vi "Path-Move.vi"(6 "Move Time":u32=500, 7 "Maze Display Ref":refnum<vi>, 8 "error in (no error)":errorcluster, 9 "Tile Array":T2[][](array[typedef]), 10 "Start":T1, 11 "Finish":T1) -> (0 "error out":errorcluster)   [LabVIEW 2020]
doc: "<B>Description:</B> Moves a colored tile through the maze.\n\n<B>Date:</B> 06/2019\n<B>Author:</B> Luke Jarocki, Choose Movement Consulting, LLC"
uses:
  Controls/TileColor.ctl
  Controls/Parse-(X,Y).ctl
panel:
  in  "stop":bool
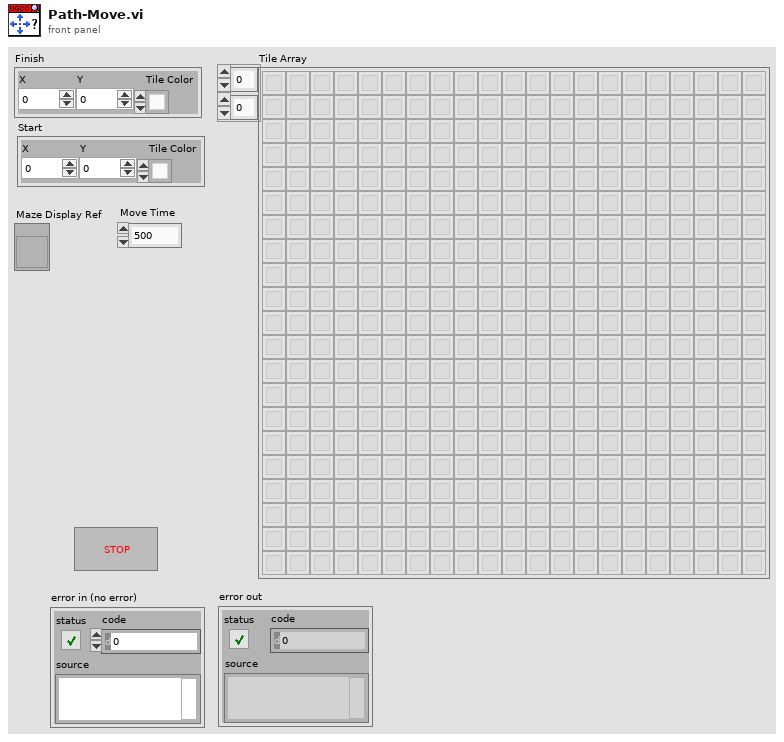
[diagram p1: front panel]
types:
  T1 = typedef "Parse-(X,Y).ctl" = cluster{"X":i32, "Y":i32, "Tile Color":T2}
  T2 = typedef "TileColor.ctl" = u16
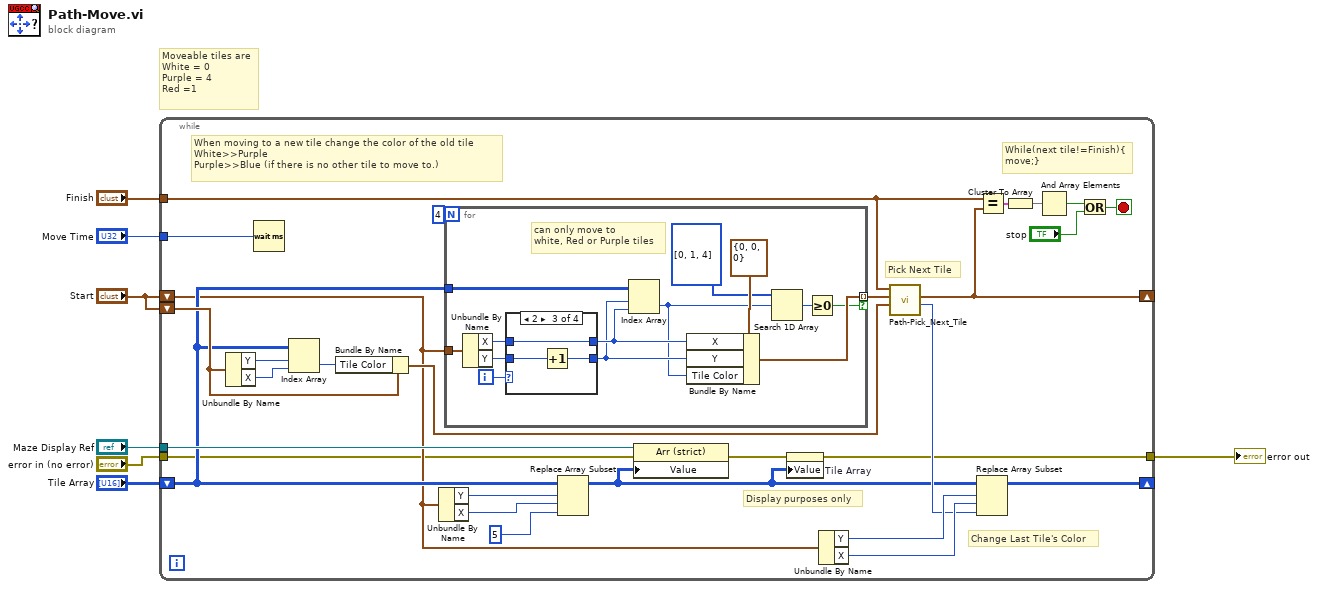
[diagram p0: block diagram]
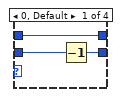
[diagram p2: hidden frame]
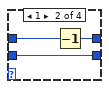
[diagram p3: hidden frame]
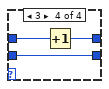
[diagram p4: hidden frame]
diagram:
  # "Moveable tiles are\nWhite = 0\nPurple = 4\nRed =1"
  n1 = while {
    tunnel: "Finish" -> [w15]
    shift-right: [w12] -> _
    shift-left: "Start" -> [w14]
    shift-right: [w33] -> _
    shift-left: "Tile Array" -> [w17]
    shift-left: "Start" -> [w25]
    tunnel: "Maze Display Ref" -> [w21]
    tunnel: "Move Time" -> [w20]
    tunnel: [w8] -> w2
    tunnel: "error in (no error)" -> [w11]
    stop <- w26 stop-if-true
    # "Change Last Tile's Color"
    # "When moving to a new tile change the color of the old tile\nWhite>>Purple\nPurple>>Blue (if there is no other tile to move to.)"
    # "While(next tile!=Finish){\nmove;}"
    # "Display purposes only"
    # "Pick Next Tile"
    n2 = Unbundle By Name(w25) -> ("Y"=w24:i32, "X"=w23:i32)
    n3 = Wait (ms)(milliseconds to wait=w20) -> ()  [unwired: 1 out]
    n4 = Index Array(array=w17, index (row)=w24, index (col)=w23) -> (element=w22:T2)
    n5 = Bundle By Name(cluster=w25, "Tile Color"=w22) -> (w16:T1)
    n6 = Unbundle By Name(w14) -> ("Y"=w19:i32, "X"=w18:i32)
    n7 = for {
      N: 4 -> [_]
      tunnel: w14 -> [w47]
      tunnel: w17 -> [w48]
      tunnel: [w43] -> w35 mode=indexing if=w37
      i -> [w49]
      # "can only move to\nwhite, Red or Purple tiles"
      n8 = Unbundle By Name(w47) -> ("X"=w46:i32, "Y"=w45:i32)
      n9 = case shown="2" w49 {
        tunnel: [w51 w54 w56 w59] -> w42
        tunnel: [w52 w53 w57 w60] -> w41
        tunnel: w46 -> [w51 w55 w56 w61]
        tunnel: w45 -> [w50 w53 w58 w60]
        frame 0, Default {
          n10 = Decrement(x=w50) -> (x-1=w52:i32)
        }
        frame 1 {
          n11 = Decrement(x=w55) -> (x-1=w54:i32)
        }
        frame 2 {
          n12 = Increment(x=w58) -> (x+1=w57:i32)
        }
        frame 3 {
          n13 = Increment(x=w61) -> (x+1=w59:i32)
        }
      }
      n14 = Index Array(array=w48, index (row)=w41, index (col)=w42) -> (element=w39:T2)
      n15 = Bundle By Name(cluster=T1 {"X"=0, "Y"=0, "Tile Color"=0} ("(X,Y)"), "X"=w42, "Y"=w41, "Tile Color"=w39) -> (w43:T1)
      n16 = Search 1D Array(1D array=T2[] [0, 1, 4], element=w39) -> (index of element=w38:i32)  [unwired: 1 in]
      n17 = Greater Or Equal To 0?(x=w38) -> (x >= 0?=w37:bool)
    }
    n18 = Replace Array Subset(array=w17, new element=T2 5 ("new element/subarray"), index (row)=w19, index (col)=w18) -> (w10:T2[][])
    n19 = property class="Arr (strict)"(reference=w21, error in=w11, "Value"=w10) -> (error out=w9:errorcluster)  [unwired: 1 out]
    n20 = property on="Tile Array" class="Arr (strict)"(error in=w9, "Value"=w10) -> (error out=w8:errorcluster)  [unwired: 1 in, 1 out]
    n21 = Unbundle By Name(w14) -> ("Y"=w32:i32, "X"=w31:i32)
    n22 = call "Path-Pick_Next_Tile.vi"("Last Tile"=w16, "Adjacent Tiles"=w35, "Goal"=w15) -> ("Tile"=w13:T2, "New Position"=w12:T1)  [unwired: 7 in]
    n23 = Replace Array Subset(array=w10, new element=w13, index (row)=w32, index (col)=w31) -> (w33:T2[][])
    n24 = Equal?(x=w15, y=w12) -> (x = y?=w30:cluster{"X":bool, "Y":bool, "Tile Color":bool})
    n25 = Cluster To Array(cluster=w30) -> (array=w29:bool[])
    n26 = And Array Elements(Boolean array=w29) -> (logical AND=w28:bool)
    n27 = Or(x=w28, y="stop") -> (x .or. y?=w26:bool)
  }
  "error out" <- w2
